vi "Test State History.vi"() -> ()   [LabVIEW 2019, in "Instrument.lvlib" / "Instrument.lvclass"]
uses:
  Instrument.lvclass
  <vilib>/dlg_ctls.llb/Space Constant.vi
  <vilib>/AdvancedString/1D String Array to Delimited String.vi
panel:
  out "Waveform Graph":dbl[](graph)
  out "x-y":dbl format="%#_6p"
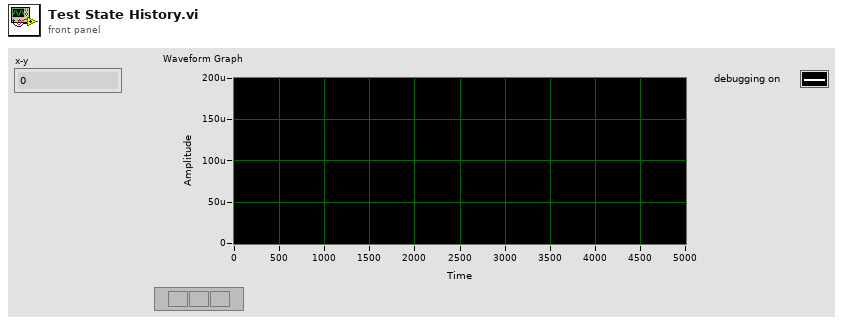
[diagram p1: front panel]
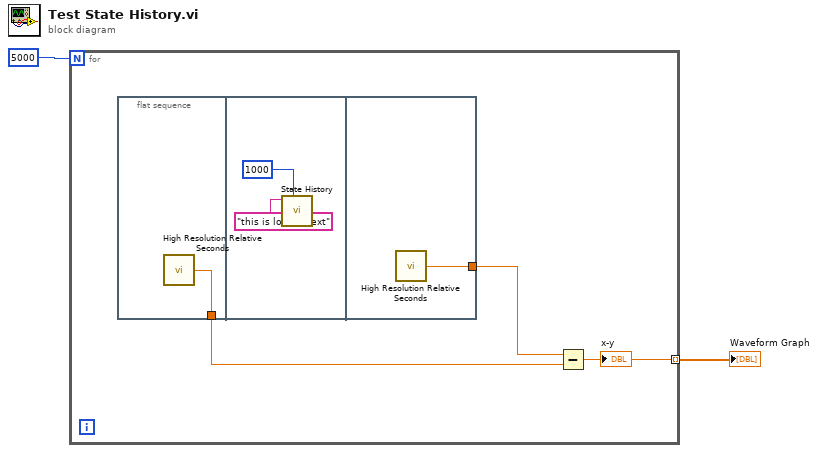
[diagram p0: block diagram]
diagram:
  n1 = for {
    N: 5000 ("history length (100)") -> [_]
    tunnel: [w3] -> w1 mode=indexing
    n2 = flat-sequence {
      tunnel: [w6] -> w4
      tunnel: [w9] -> w5
      frame #0 {
        n3 = call <vilib>:"High Resolution Relative Seconds.vi"() -> ("relative seconds"=w6:dbl)
      }
      frame #1 {
        n4 = call "State History.vi"("history length (100)"=1000, "Current State"="this is longer text") -> ()  [unwired: 9 in, 1 out]
      }
      frame #2 {
        n5 = call <vilib>:"High Resolution Relative Seconds.vi"() -> ("relative seconds"=w9:dbl)
      }
    }
    n6 = Subtract(x=w5, y=w4) -> (x-y=w3:dbl)
    "x-y" <- w3
  }
  "Waveform Graph" <- w1
